vi "LoadConfigFile.vi"(7 "error in (no error)":errorcluster) -> (15 "FTP password":string, 16 "Licensee":string, 17 "FTP user":string, 18 "Key":string, 19 "Use FTP":bool, 20 "IP":string caption="Robot IP Address", 21 "RoboguideRobotPath":path, 22 "ConnectRoboguide":bool, 23 "Use Telnet":bool, 24 "Telnet password":string, 25 "Use SNPX":bool, 27 "error out":errorcluster)   [LabVIEW 2017]
uses:
  <vilib>/Utility/config.llb/NI_LVConfig.lvlib
  <vilib>/Utility/config.llb/Read Key (Boolean).vi
  <vilib>/Utility/config.llb/Read Key (String).vi
  <vilib>/Utility/config.llb/Read Key (Path).vi
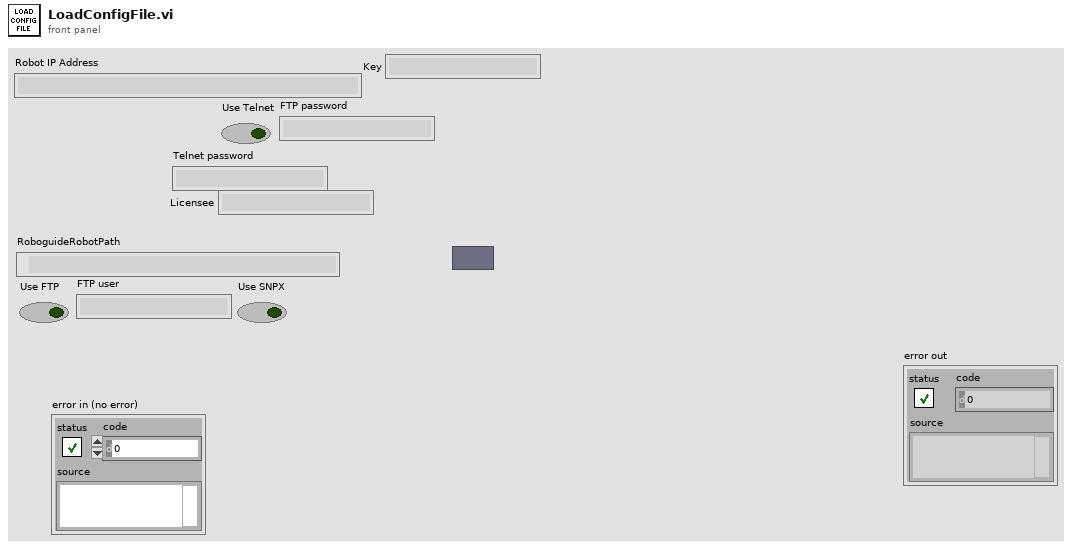
[diagram p1: front panel]
types:
  T1 = typedef "NI_LVConfig.lvlib/Config Data RefNum.ctl" = refnum<k1>
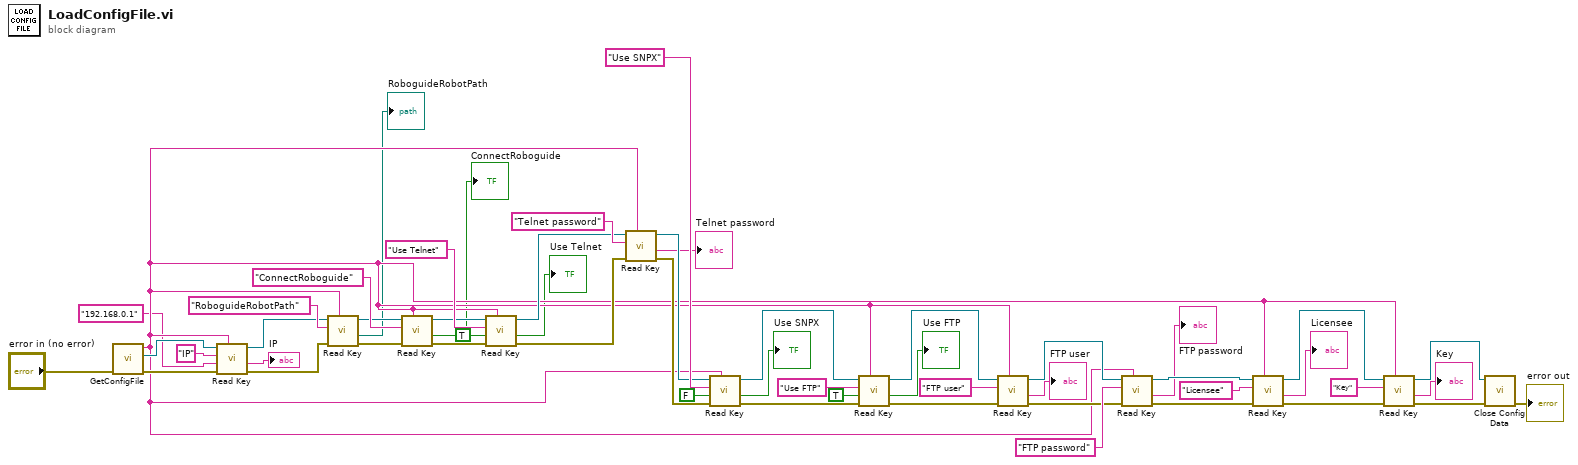
[diagram p0: block diagram]
diagram:
  n1 = call "GetConfigFile.vi"("error in (no error)"="error in (no error)") -> ("error out"=w52:errorcluster, "refnum"=w51:T1, "section"=w19:string)  [unwired: 8 in]
  n2 = call-poly <vilib>:"Read Key.vi"("section"=w19, "error in (no error)"=w52, "default value"="192.168.0.1", "key"="IP", "refnum"=w51) -> ("error out"=w31:errorcluster, "value"=→"IP":string, "refnum out"=w17:T1)  [unwired: 3 in, 1 out]
  n3 = call-poly <vilib>:"Read Key.vi"("section"=w19, "error in (no error)"=w31, "key"="RoboguideRobotPath", "refnum"=w17) -> ("error out"=w30:errorcluster, "value"=→"RoboguideRobotPath":path, "refnum out"=w18:T1)  [unwired: 4 in, 1 out]
  n4 = call-poly <vilib>:"Read Key.vi"("section"=w19, "error in (no error)"=w30, "key"="ConnectRoboguide", "refnum"=w18) -> ("error out"=w29:errorcluster, "value"=→"ConnectRoboguide":bool, "refnum out"=w32:T1)  [unwired: 4 in, 1 out]
  n5 = call-poly <vilib>:"Read Key.vi"("section"=w19, "error in (no error)"=w29, "default value"=TRUE, "key"="Use Telnet", "refnum"=w32) -> ("error out"=w28:errorcluster, "value"=→"Use Telnet":bool, "refnum out"=w33:T1)  [unwired: 3 in, 1 out]
  n6 = call-poly <vilib>:"Read Key.vi"("section"=w19, "error in (no error)"=w28, "key"="Telnet password", "refnum"=w33) -> ("error out"=w27:errorcluster, "value"=→"Telnet password":string, "refnum out"=w34:T1)  [unwired: 4 in, 1 out]
  n7 = call-poly <vilib>:"Read Key.vi"("section"=w19, "error in (no error)"=w27, "default value"=FALSE, "key"="Use SNPX", "refnum"=w34) -> ("error out"=w26:errorcluster, "value"=→"Use SNPX":bool, "refnum out"=w35:T1)  [unwired: 3 in, 1 out]
  n8 = call-poly <vilib>:"Read Key.vi"("section"=w19, "error in (no error)"=w26, "default value"=TRUE, "key"="Use FTP", "refnum"=w35) -> ("error out"=w25:errorcluster, "value"=→"Use FTP":bool, "refnum out"=w36:T1)  [unwired: 3 in, 1 out]
  n9 = call-poly <vilib>:"Read Key.vi"("section"=w19, "error in (no error)"=w25, "key"="FTP user", "refnum"=w36) -> ("error out"=w24:errorcluster, "value"=→"FTP user":string, "refnum out"=w37:T1)  [unwired: 4 in, 1 out]
  n10 = call-poly <vilib>:"Read Key.vi"("section"=w19, "error in (no error)"=w24, "key"="FTP password", "refnum"=w37) -> ("error out"=w23:errorcluster, "value"=→"FTP password":string, "refnum out"=w38:T1)  [unwired: 4 in, 1 out]
  n11 = call-poly <vilib>:"Read Key.vi"("section"=w19, "error in (no error)"=w23, "key"="Licensee", "refnum"=w38) -> ("error out"=w22:errorcluster, "value"=→"Licensee":string, "refnum out"=w39:T1)  [unwired: 4 in, 1 out]
  n12 = call-poly <vilib>:"Read Key.vi"("section"=w19, "error in (no error)"=w22, "key"="Key", "refnum"=w39) -> ("error out"=w21:errorcluster, "value"=→"Key":string, "refnum out"=w40:T1)  [unwired: 4 in, 1 out]
  n13 = call <vilib>:"Close Config Data.vi"("error in (no error)"=w21, "refnum"=w40) -> ("error out"=→"error out":errorcluster)  [unwired: 8 in, 1 out]
